vi "Verify File.vi"(4 "Execution time (s)":dbl=-1.0, 5 "Assert Only? (F)":bool, 6 "error code (1)":i32=1, 7 "Options":refnum<class "Options.lvclass">, 8 "error in":errorcluster, 10 "path to file":path, 11 "Label":string) -> (0 "error out":errorcluster, 2 "Properties":refnum<class "Properties.Assert.lvclass">)   [LabVIEW 2020, in "Caraya.Extension.lvlib"]
doc: "Takes in a file path. In general compares to approved using the filehash. If it detects a .vi or .ctl file, it uses the built-in comparison function in LabVIEW. In LabVIEW 2020, It is buggy. Apparently some of those bugs have been fixed in newer versions."
uses:
  Caraya.Extension.lvlib
  Approval Tests/Options/Options.lvclass
  <vilib>/addons/_JKI Toolkits/Caraya/classes/Properties.Assert/Properties.Assert.lvclass
  Approval Tests/Options/Options.lvclass/Options.ctl
  Approval Tests/Naming Data/Naming Data.lvclass/Naming Data.ctl
  <vilib>/addons/_JKI Toolkits/Caraya/classes/Assert/Assert.lvclass
  Approval Tests/Approval Tests.lvlib
  <vilib>/addons/_JKI Toolkits/Caraya/classes/Assert/Assert True.vi
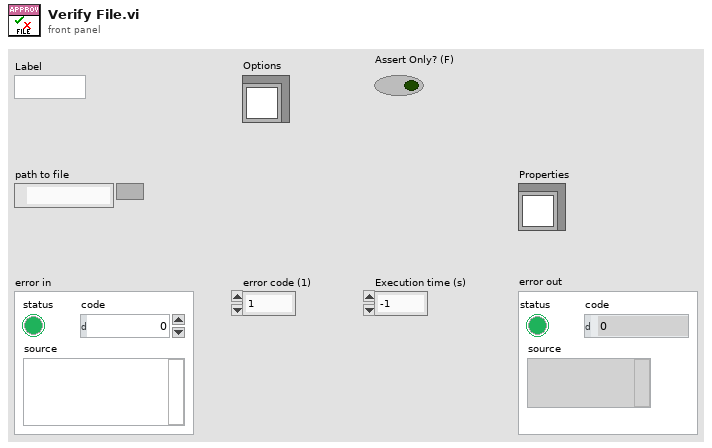
[diagram p1: front panel]
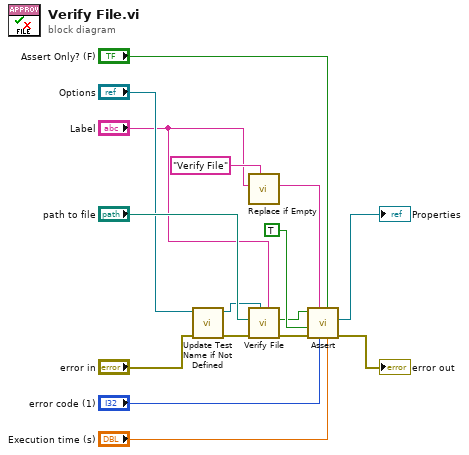
[diagram p0: block diagram]
diagram:
  n1 = call "Update Test Name if Not Defined.vi"("error in"="error in", "Options in"="Options") -> ("error out"=w13:errorcluster, "Options out"=w4:refnum<class "Options.lvclass">)  [unwired: 8 in]
  n2 = call "Replace if Empty.vi"("if empty"="Verify File" ("Label"), "Text in"="Label") -> ("Text out"=w1:string)  [unwired: 9 in]
  n3 = call "Verify File.vi"("Label"="Label", "Options"=w4, "error in"=w13, "Path to Binary File to Verify"="path to file") -> ("error out"=w14:errorcluster, "Passed?"=w11:bool)  [unwired: 5 in, 1 out]
  n4 = call-poly <vilib>:"Assert.vi"("Execution time (s)"="Execution time (s)", "Assert Only? (F)"="Assert Only? (F)", "error code (1)"="error code (1)", "Label"=w1, "error in (no error)"=w14, "Register with caller test (F)"=TRUE, "True?"=w11) -> ("error out"=→"error out":errorcluster, "Properties"=→"Properties":refnum<class "Properties.Assert.lvclass">)  [unwired: 3 in]
